vi "Paint_Tracks_Before-After-4.vi"(5 "[IN] Number of event":i8=2, 6 "[IN] Localization Settings":T4 {"[IN] Image Type" items=["Grayscale (U8)", "Grayscale (I16)", "Grayscale (SGL)", "Complex (CSG)", "RGB (U32)", "HSL (U32)", "RGB (U64)", "Grayscale (U16)"]; "[IN] Particle Filter Setups"."Type of particle filter"."Measurement Parameter" items=["Center of Mass X", "Center of Mass Y", "First Pixel X", "First Pixel Y", "Bounding Rect Left", "Bounding Rect Top", "Bounding Rect Right", "Bounding Rect Bottom", "Max Feret Diameter Start X", "Max Feret Diameter Start Y", "Max Feret Diameter End X", "Max Feret Diameter End Y", "Max Horiz. Segment Length Left", "Max Horiz. Segment Length Right", "Max Horiz. Segment Length Row", "-", "Bounding Rect Width", "Bounding Rect Height", "Bounding Rect Diagonal", "Perimeter", "Convex Hull Perimeter", "Holes' Perimeter", "Max Feret Diameter", "Equivalent Ellipse Major Axis", "Equivalent Ellipse Minor Axis", "Equivalent Ellipse Minor Axis (Feret)", "Equivalent Rect Long Side", "Equivalent Rect Short Side", "Equivalent Rect Diagonal", "Equivalent Rect Short Side (Feret)", "Average Horiz. Segment Length", "Average Vert. Segment Length", "Hydraulic Radius", "Waddel Disk Diameter", "-", "Area", "Holes' Area", "Particle & Holes' Area", "Convex Hull Area", "Image Area", "-", "Number of Holes", "Number of Horiz. Segments", "Number of Vert. Segments", "-", "Orientation", "Max Feret Diameter Orientation", "-", "% Area/Image Area", "% Area/(Particle & Holes' Area)", "Ratio of Equivalent Ellipse Axes", "Ratio of Equivalent Rect Sides", "-", "Elongation Factor", "Compactness Factor", "Heywood Circularity Factor", "Type Factor", "-", "Sum X", "Sum Y", "Sum XX", "Sum XY", "Sum YY", "Sum XXX", "Sum XXY", "Sum XYY", "Sum YYY", "-", "Moment of Inertia XX", "Moment of Inertia XY", "Moment of Inertia YY", "Moment of Inertia XXX", "Moment of Inertia XXY", "Moment of Inertia XYY", "Moment of Inertia YYY", "Norm. Moment of Inertia XX", "Norm. Moment of Inertia XY", "Norm. Moment of Inertia YY", "Norm. Moment of Inertia XXX", "Norm. Moment of Inertia XXY", "Norm. Moment of Inertia XYY", "Norm. Moment of Inertia YYY", "Hu Moment 1", "Hu Moment 2", "Hu Moment 3", "Hu Moment 4", "Hu Moment 5", "Hu Moment 6", "Hu Moment 7"]}, 7 "[IN] Images Array":T5[](array[typedef]), 8 "error IN":errorcluster, 10 "[IN] Grouped Tracks Values":T6) -> (0 "error OUT":errorcluster, 2 "[OUT] Image with\nDisplacements":T5)   [LabVIEW 2013]
doc: "Drawing of grouped tracks on the LoG processed frame"
uses:
  <vilib>/vision/Image Controls.llb/IMAQ Image.ctl
  <vilib>/vision/Avi.llb/IMAQ AVI2 Refnum.ctl
panel:
  in  "[IN] Additional Index":i32
  in  "[IN] Delete Tracs":bool
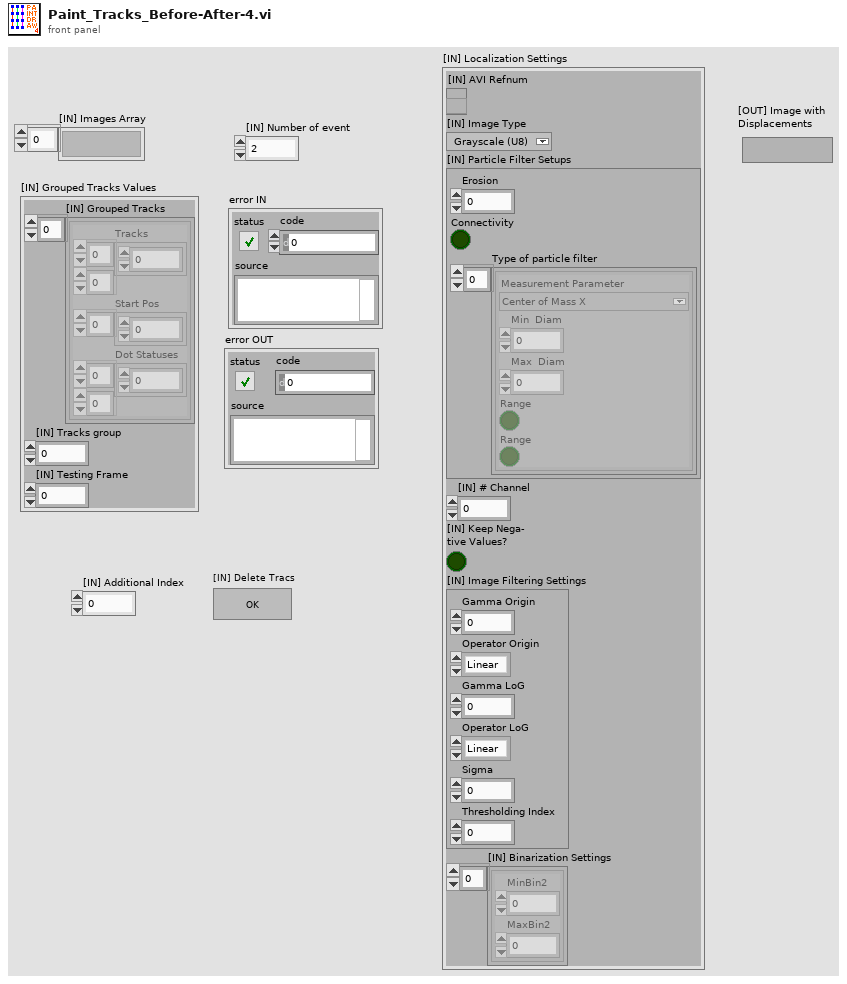
[diagram p1: front panel]
types:
  T1 = typedef "IMAQ AVI2 Refnum.ctl" = refnum<k20>
  T2 = typedef "Image Type" = u32
  T3 = typedef "Particle Parameters" = i32
  T4 = cluster{"[IN] AVI Refnum":T1, "[IN] Image Type":T2, "[IN] Particle Filter Setups":cluster{"Erosion":i32, "Connectivity ":bool, "Type of particle filter":cluster{"Measurement Parameter":T3, "Min  Diam":dbl, "Max  Diam":dbl, "Range":bool, "Range":bool}[]}, "[IN] # Channel":u8, "[IN] Keep Nega-\ntive Values?":bool, "[IN] Image Filtering Settings":cluster{"Gamma Origin":sgl, "Operator Origin":enum32{"Linear", "Log", "Exp", "Square", "Square root", "Power X", "Power 1/X"}, "Gamma LoG":sgl, "Operator LoG":enum32{"Linear", "Log", "Exp", "Square", "Square root", "Power X", "Power 1/X"}, "Sigma":dbl, "Thresholding Index":i8}, "[IN] Binarization Settings":cluster{"MinBin2":sgl, "MaxBin2":sgl}[]}
  T5 = typedef "IMAQ Image.ctl" = refnum<image>
  T6 = cluster{"[IN] Grouped Tracks":cluster{"Tracks":dbl[][], "Start Pos":i32[], "Dot Statuses":i16[][]}[], "[IN] Tracks group":i32, "[IN] Testing Frame ":u32}
  T7 = cluster{"Tracks":dbl[][], "Start Pos":i32[], "Dot Statuses":i16[][]}[]
  T8 = cluster{"Tracks":dbl[][], "Start Pos":i32[], "Dot Statuses":i16[][]}
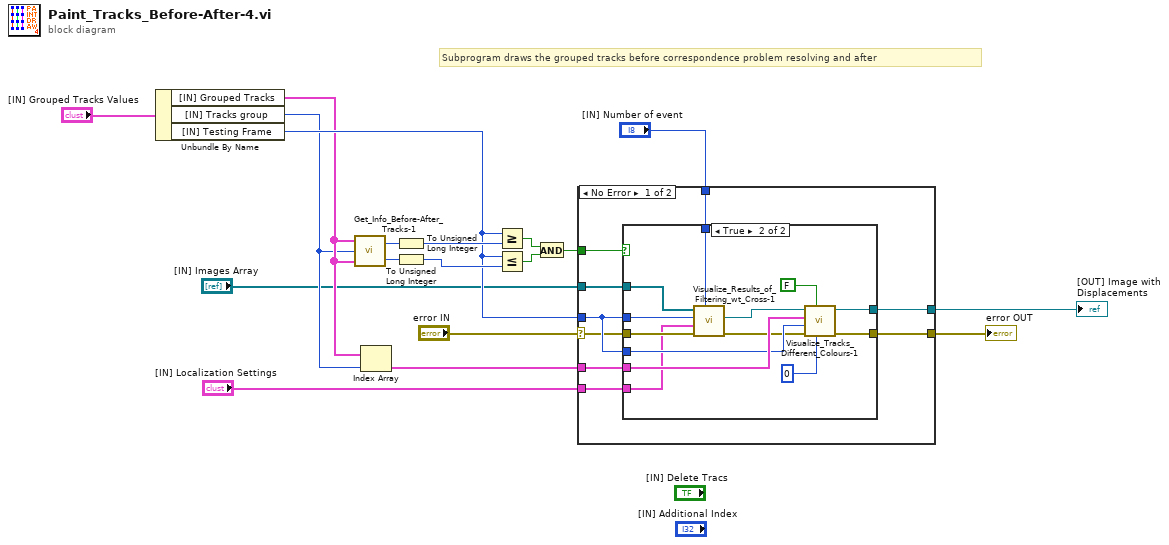
[diagram p0: block diagram]
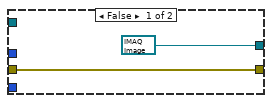
[diagram p2: hidden frame]
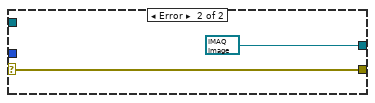
[diagram p3: hidden frame]
diagram:
  # "Subprogram draws the grouped tracks before correspondence problem resolving and after"
  n1 = Unbundle By Name("[IN] Grouped Tracks Values") -> ("[IN] Grouped Tracks"=w6:T7, "[IN] Tracks group"=w5:i32, "[IN] Testing Frame"=w7:u32)
  n2 = call "Get_Info_Before-After_Tracks-1.vi"("[IN] After Tracks"=w6, "[IN] Tracks group"=w5, "[IN] Before Tracks"=w6) -> ("[OUT] Maximal Frame\n(finish point all tracks)"=w16:i32, "[OUT] Min Start Pos"=w18:i32)
  n3 = Index Array(array=w6, index=w5) -> (element=w11:T8)
  n4 = To Unsigned Long Integer(number=w18) -> (unsigned 32bit integer=w17:u32)
  n5 = To Unsigned Long Integer(number=w16) -> (unsigned 32bit integer=w15:u32)
  n6 = Greater Or Equal?(x=w7, y=w17) -> (x >= y?=w14:bool)
  n7 = Less Or Equal?(x=w7, y=w15) -> (x <= y?=w13:bool)
  n8 = And(x=w14, y=w13) -> (x .and. y?=w12:bool)
  n9 = case shown="No Error" "error IN" {
    selector: "error IN" -> [w22 w44]
    tunnel: w12 -> [w27 _]
    tunnel: w11 -> [w26 _]
    tunnel: [w25 w44] -> w10
    tunnel: [w24 T5 refnum ("[OUT] Image with\nDisplacements")] -> w9
    tunnel: w7 -> [w23 _]
    tunnel: "[IN] Number of event" -> [w21 _]
    tunnel: "[IN] Images Array" -> [w20 _]
    tunnel: "[IN] Localization Settings" -> [w19 _]
    frame No Error {
      n10 = case shown="True" w27 {
        tunnel: w23 -> [_ w37]
        tunnel: w26 -> [_ w42]
        tunnel: w23 -> [_ w41]
        tunnel: [T5 refnum ("[OUT] Image with\nDisplacements") w40] -> w24
        tunnel: [w29 w39] -> w25
        tunnel: w22 -> [w29 w36]
        tunnel: w21 -> [_ w35]
        tunnel: w20 -> [_ w34]
        tunnel: w19 -> [_ w31]
        frame False {
        }
        frame True {
          n11 = call "Visualize_Results_of_Filtering_wt_Cross-1.vi"("[IN] Number of event"=w35, "error IN"=w36, "[IN] Localization Settings"=w31, "# Frame"=w37, "[IN] Images Array"=w34) -> ("error OUT"=w32:errorcluster, "[OUT] LoG with Particles"=w33:T5)  [unwired: 5 in]
          n12 = call "Visualize_Tracks_Different_Colours-1.vi"("[IN] Additional Index"=0, "[IN] Delete Tracs"=FALSE, "error IN"=w32, "[IN] Testing Frame"=w41, "[IN] Tracks"=w42, "[IN] LoG Pro-\ncessed Image"=w33) -> ("error OUT"=w39:errorcluster, "[OUT] Image with\nDisplacements"=w40:T5)  [unwired: 2 in]
        }
      }
    }
    frame Error {
    }
  }
  "error OUT" <- w10
  "[OUT] Image with\nDisplacements" <- w9
